vi "Pockels Cal-Initialise ring and listbox26_01_18.vi"(7 "Function":T1(ring), 8 "error in (no error)":errorcluster, 10 "Cal Wav listbox":refnum<vi>, 11 "Cal files listbox":refnum<vi>) -> (0 "error out":errorcluster, 3 "All data loaded":string[][](array[string]))   [LabVIEW 2020]
uses:
  Typedefs/Which path.ctl
  <userlib>/My Palettes.lib/Files & paths/Spreadsheet/Read From Spreadsheet File (string)-Mod.vi
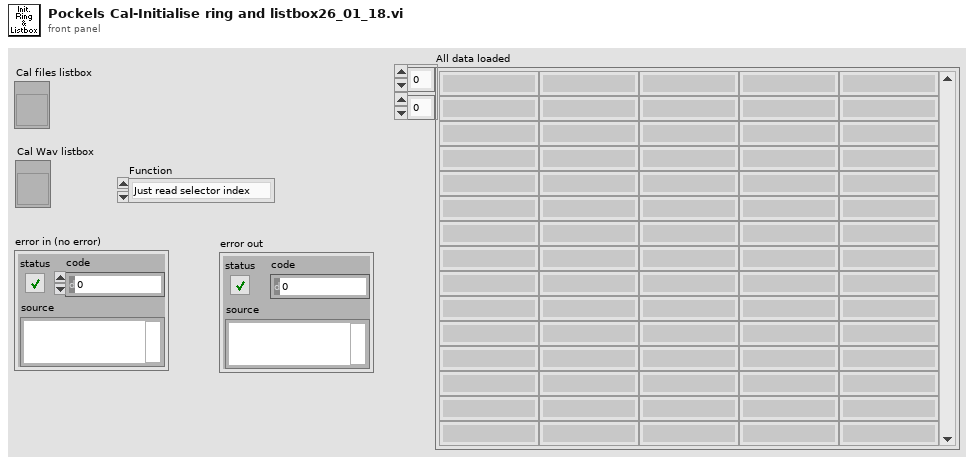
[diagram p1: front panel]
types:
  T1 = enum16{"Just read selector index", "remap to selected cal", "map to active cal"}
  T2 = typedef "Which path.ctl" = enum16{"Configuration Files", "Calibration Files", "Images", "Setup.ini", "Loaded User profile.ini", "User's-Previous session.ini", "New user profile.ini", "Selected User profile.ini", "User profiles folder", "Power meter scaling.txt", "FOV Cal.ini", "Calibration.ini"}
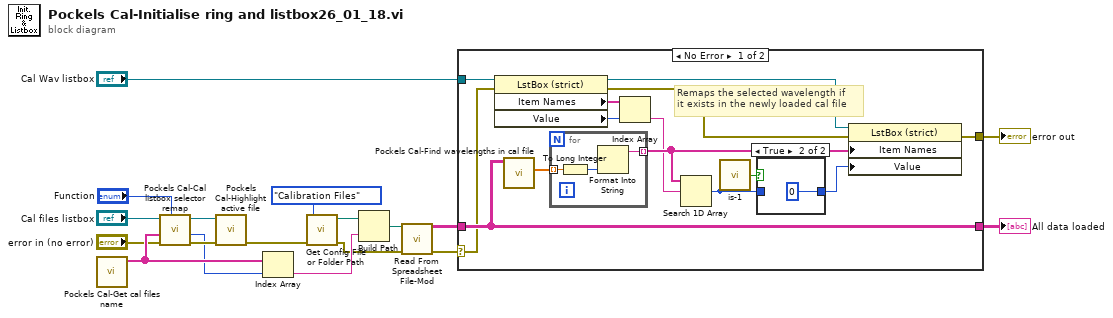
[diagram p0: block diagram]
diagram:
  n1 = call "Pockels Cal-Get cal files name.vi"() -> ("Filtered Array out"=w15:string[])  [unwired: 11 in]
  n2 = call "Pockels Cal-Cal listbox selector remap.vi"("Function"="Function", "error in (no error)"="error in (no error)", "Filtered Array in"=w15, "ListBox in"="Cal files listbox") -> ("error out"=w4:errorcluster, "index of element"=w2:i32, "ListBox out"=w1:refnum<vi>)  [unwired: 5 in]
  n3 = call "Pockels Cal-Highlight active file.vi"("error in (no error)"=w4, "ListBox in"=w1) -> ("error out"=w3:errorcluster)  [unwired: 9 in]
  n4 = Index Array(array=w15, index=w2) -> (element=w8:string)
  n5 = call "Get Config File or Folder Path.vi"("Error In"=w3, "Which file or folder?"=Which_path."Calibration Files" ("Which path?")) -> ("Error Out"=w7:errorcluster, "File Path"=w12:path)  [unwired: 7 in, 1 out]
  n6 = Build Path(base path=w12, name or relative path=w8) -> (appended path=w11:path)
  n7 = call-poly <userlib>:"Read From Spreadsheet File-Mod.vi"("file path (dialog if empty)"=w11, "error in"=w7) -> ("all rows"=w10:string[][], "error out"=w9:errorcluster)  [unwired: 8 in, 4 out]
  n8 = case shown="No Error" w9 {
    selector: w9 -> [w20 w38]
    tunnel: w10 -> [w31 _]
    tunnel: [w31 _] -> w17
    tunnel: [w30 w38] -> w18
    tunnel: "Cal Wav listbox" -> [w27 _]
    frame No Error {
      # "Remaps the selected wavelength if \nit exists in the newly loaded cal file"
      n9 = property on="Property Node" class="LstBox (strict)"(reference=w27, error in=w20) -> (reference out=w26:refnum<vi>, error out=w19:errorcluster, "Item Names"=w29:string[], "Value"=w28:i32)
      n10 = call "Pockels Cal-Find wavelengths in cal file.vi"("Loaded cal file"=w31) -> ("Pockels cal'd wavelengths"=w32:dbl[])  [unwired: 9 in, 1 out]
      n11 = for {
        tunnel: w32 -> [w37] mode=indexing
        tunnel: [w36] -> w25 mode=indexing
        n12 = To Long Integer(number=w37) -> (32bit integer=w35:i32)
        n13 = Format Into String(w35) -> (resulting string=w36:string)  [unwired: 3 in, 1 out]
      }
      n14 = Index Array(array=w29, index=w28) -> (element=w24:string)
      n15 = Search 1D Array(1D array=w25, element=w24) -> (index of element=w21:i32)  [unwired: 1 in]
      n16 = call "is-1.vi"("Value"=w21) -> ("is -1?"=w23:bool)  [unwired: 4 in]
      n17 = case shown="True" w23 {
        tunnel: [w33 0] -> w22
        tunnel: w21 -> [w33 _]
        frame False {
        }
        frame True {
        }
      }
      n18 = property on="Property Node" class="LstBox (strict)"(reference=w26, error in=w19, "Item Names"=w25, "Value"=w22) -> (error out=w30:errorcluster)  [unwired: 1 out]
    }
    frame Error {
    }
  }
  "error out" <- w18
  "All data loaded" <- w17
